vi "toggle Plunger.vi"(7 "Plunger":T2(ring), 8 "error in (no error)":errorcluster) -> (0 "error out":errorcluster)   [LabVIEW 2013]
panel:
  out "cluster":T1
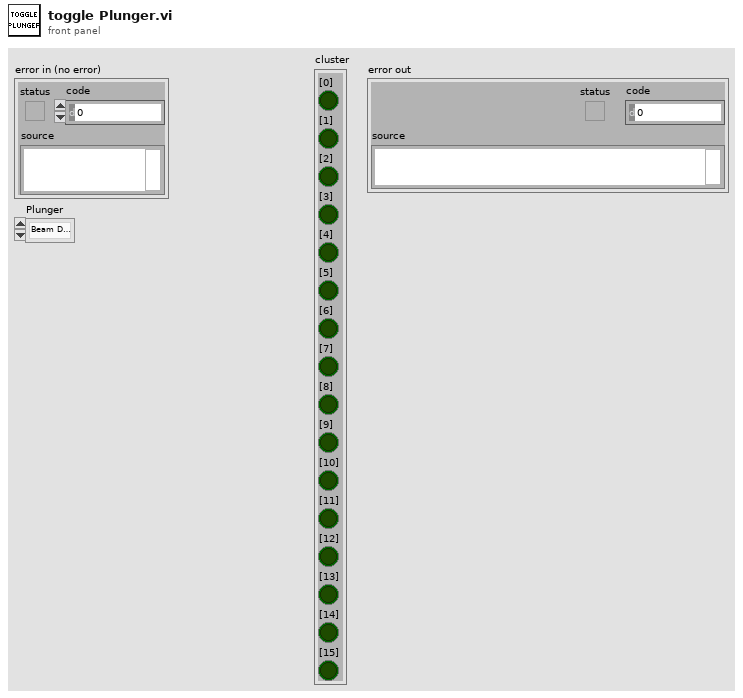
[diagram p1: front panel]
types:
  T1 = cluster{"[0]":bool, "[1]":bool, "[2]":bool, "[3]":bool, "[4]":bool, "[5]":bool, "[6]":bool, "[7]":bool, "[8]":bool, "[9]":bool, "[10]":bool, "[11]":bool, "[12]":bool, "[13]":bool, "[14]":bool, "[15]":bool}
  T2 = enum16{"Beam Dump 1", "Beam Dump 2", "Wedge", "Phosphor"}
  T3 = cluster{bool, bool, bool, bool, bool, bool, bool, bool, bool, bool, bool, bool, bool, bool, bool, bool}
  T4 = cluster{cluster{bool, bool, bool, bool, bool, bool, bool, bool, bool, bool, bool, bool, bool, bool, bool, bool}, cluster{bool, bool, bool, bool, bool, bool, bool, bool, bool, bool, bool, bool, bool, bool, bool, bool}}
  T5 = enum16{"Read", "Write", "ReadWrite", "BufferedRead", "BufferedReadWrite"}
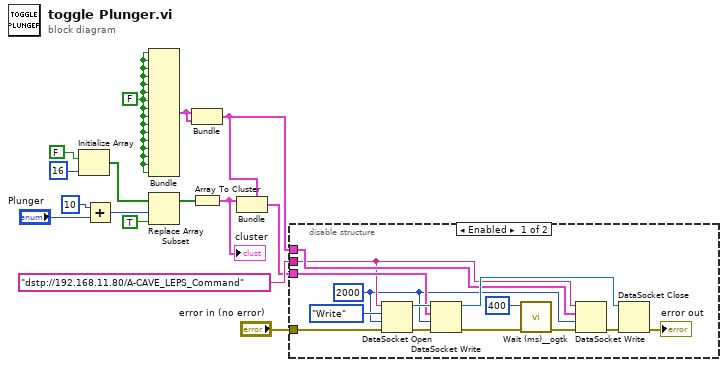
[diagram p0: block diagram]
diagram:
  w2 = FALSE
  n1 = Initialize Array(FALSE, 16 ("dimension size")) -> (w13:bool[])
  n2 = Add(x=10, y="Plunger") -> (x+y=w11:i32)
  n3 = Bundle(w2, w2, w2, w2, w2, w2, w2, w2, w2, w2, w2, w2, w2, w2, w2, w2) -> (w3:T3)  [unwired: 1 in]
  n4 = Replace Array Subset(array=w13, new element=TRUE ("new element/subarray"), index=w11) -> (w9:bool[])
  n5 = Bundle(w3, w3) -> (w1:T4)  [unwired: 1 in]
  n6 = Array To Cluster(array=w9) -> (cluster=w8:T1)
  "cluster" <- w8
  n7 = Bundle(cluster=w1, w8) -> (w6:T4)  [unwired: 1 in]
  n8 = disable-structure shown="Enabled" {
    disable-tunnel: "dstp://192.168.11.80/A-CAVE_LEPS_Command" ("Target_URL 2") -> [w20 _]
    disable-tunnel: w6 -> [w25 _]
    disable-tunnel: "error in (no error)" -> [w23 _]
    disable-tunnel: w1 -> [w21 _]
    frame Enabled {
      w19 = 2000 ("ms timeout (10000)")
      n9 = DataSocket Open(8:w23, 9:w19, 10:T5."Write" ("mode"), 11:w20) -> (0:w29:errorcluster, 3:w27:refnum<k13>)
      n10 = DataSocket Write(8:w29, 9:w19, 10:w25, 11:w27) -> (0:w18:errorcluster, 3:w28:refnum<k13>)  [unwired: 1 out]
      n11 = call <userlib>:"Wait (ms)__ogtk.vi"("error in (no error)"=w18, "milliseconds to wait"=u32 400) -> ("error out"=w17:errorcluster)  [unwired: 8 in, 1 out]
      n12 = DataSocket Write(8:w17, 9:w19, 10:w21, 11:w20) -> (0:w22:errorcluster)  [unwired: 2 out]
      n13 = DataSocket Close(8:w22, 11:w28) -> (0:→"error out":errorcluster)  [unwired: 1 in, 1 out]
    }
    frame Disabled {
    }
  }
